vi "SubVIs1.vi"(10 "B":dbl[](array[numeric]), 11 "A":dbl[](array[numeric])) -> (2 "(A-B)/2":dbl[](array[numeric]), 3 "(A+B)/2":dbl[](array[numeric]))   [LabVIEW 2011]
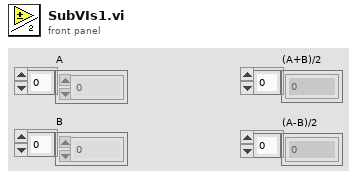
[diagram p1: front panel]
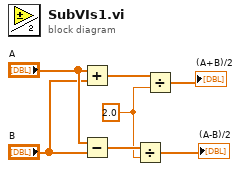
[diagram p0: block diagram]
diagram:
  w2 = 2.0
  n1 = Add(x="A", y="B") -> (x+y=w7:dbl[])
  n2 = Subtract(x="A", y="B") -> (x-y=w3:dbl[])
  n3 = Divide(x=w3, y=w2) -> (x/y=→"(A-B)/2":dbl[])
  n4 = Divide(x=w7, y=w2) -> (x/y=→"(A+B)/2":dbl[])
